vi "manage_selected_cities.vi"(8 "error in":errorcluster, 9 "selected_city":refnum<vi>, 10 "multicity":bool, 11 "Selected_cities_refs[]":refnum<vi>[](array[refnum])) -> (0 "error out":errorcluster, 3 "Selected_Cities[]":T1[](array[typedef]))   [LabVIEW 2018]
uses:
  controls/wind_turbine_icon_basic.ctl
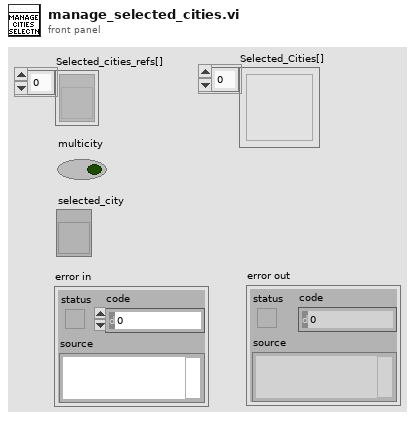
[diagram p1: front panel]
types:
  T1 = typedef "wind_turbine_icon_basic.ctl" = bool
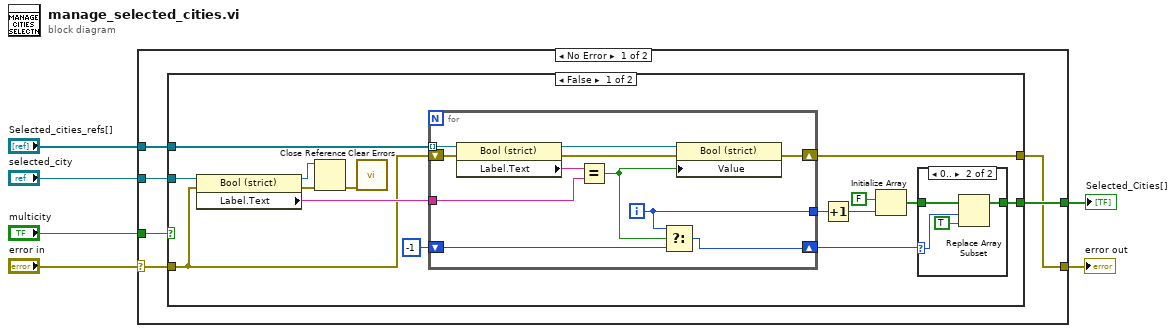
[diagram p0: block diagram]
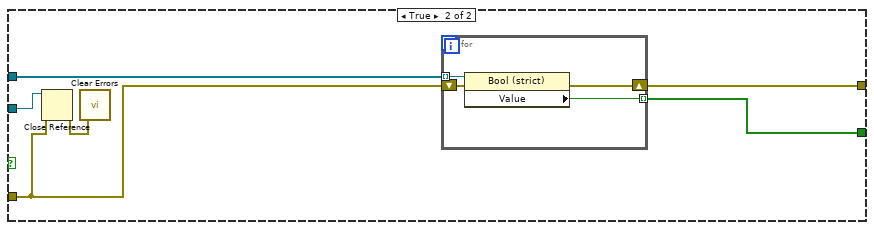
[diagram p3: hidden frame]
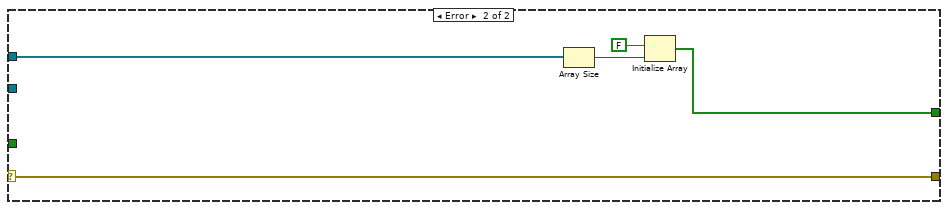
[diagram p4: hidden frame]
diagram:
  n1 = case shown="No Error" "error in" {
    selector: "error in" -> [w10 w58]
    tunnel: [w12 w54] -> w6
    tunnel: "Selected_cities_refs[]" -> [w11 w56]
    tunnel: "multicity" -> [w8 _]
    tunnel: [w9 w58] -> w2
    tunnel: "selected_city" -> [w7 _]
    frame No Error {
      n2 = case shown="False" w8 {
        tunnel: [w20 w49] -> w12
        tunnel: w11 -> [w27 w48]
        tunnel: w10 -> [w14 w44]
        tunnel: [w26 w47] -> w9
        tunnel: w7 -> [w19 w45]
        frame False {
          n3 = property class="Bool (strict)"(reference=w19, error in=w14) -> (reference out=w16:refnum<vi>, error out=w17:errorcluster, "Label.Text"=w18:string)
          n4 = Close Reference(reference=w16, error in (no error)=w17) -> (error out=w15:errorcluster)
          n5 = call <vilib>:"Clear Errors.vi"("error in (no error)"=w15) -> ()  [unwired: 5 in, 2 out]
          n6 = for {
            tunnel: w27 -> [w40] mode=indexing
            shift-right: [w34] -> w26
            shift-left: w14 -> [w39]
            shift-right: [w41] -> w13
            shift-left: -1 -> [w42]
            tunnel: [w33] -> w23
            tunnel: w18 -> [w36]
            i -> [w33]
            n7 = property class="Bool (strict)"(reference=w40, error in=w39) -> (reference out=w37:refnum<vi>, error out=w38:errorcluster, "Label.Text"=w35:string)
            n8 = Equal?(x=w35, y=w36) -> (x = y?=w43:bool)
            n9 = Select(t=w33, s=w43, f=w42) -> (s? t:f=w41:i32)
            n10 = property class="Bool (strict)"(reference=w37, error in=w38, "Value"=w43) -> (error out=w34:errorcluster)  [unwired: 1 out]
          }
          n11 = Increment(x=w23) -> (x+1=w22:i32)
          n12 = Initialize Array(FALSE, w22) -> (w21:bool[])
          n13 = case shown="0.." w13 {
            selector: w13 -> [_ w29]
            tunnel: w21 -> [w28 w32]
            tunnel: [w28 w30] -> w20
            frame -1, Default {
            }
            frame 0.. {
              n14 = Replace Array Subset(array=w32, new element=TRUE ("new element/subarray"), index=w29) -> (w30:bool[])
            }
          }
        }
        frame True {
          n15 = Close Reference(reference=w45, error in (no error)=w44) -> (error out=w46:errorcluster)
          n16 = call <vilib>:"Clear Errors.vi"("error in (no error)"=w46) -> ()  [unwired: 5 in, 2 out]
          n17 = for {
            tunnel: w48 -> [w53] mode=indexing
            tunnel: [w51] -> w49 mode=indexing
            shift-right: [w50] -> w47
            shift-left: w44 -> [w52]
            n18 = property class="Bool (strict)"(reference=w53, error in=w52) -> (error out=w50:errorcluster, "Value"=w51:T1)  [unwired: 1 out]
          }
        }
      }
    }
    frame Error {
      n19 = Array Size(array=w56) -> (size(s)=w55:i32)
      n20 = Initialize Array(FALSE, w55) -> (w54:bool[])
    }
  }
  "Selected_Cities[]" <- w6
  "error out" <- w2
